vi "DPO_7K_Set_Number_of_Averages.vi"(8 "Error In":errorcluster, 10 "Number of Waveforms":i32, 11 "VISA resource name in":refnum<visa-resource-name>) -> (0 "Error Out":errorcluster, 3 "VISA resource name out":refnum<visa-resource-name>)   [LabVIEW 2020]
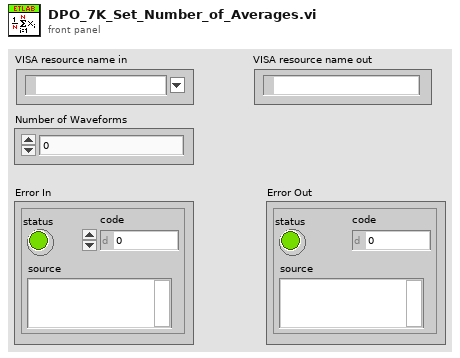
[diagram p1: front panel]
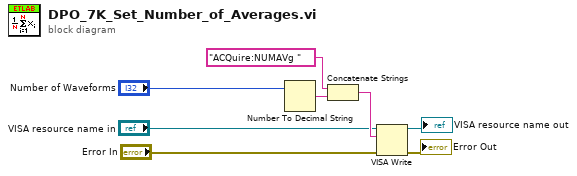
[diagram p0: block diagram]
diagram:
  n1 = Number To Decimal String(number="Number of Waveforms") -> (decimal integer string=w7:string)  [unwired: 1 in]
  n2 = Concatenate Strings("ACQuire:NUMAVg " ("write buffer"), w7) -> (w5:string)
  n3 = VISA Write(VISA resource name="VISA resource name in", write buffer=w5, error in (no error)="Error In") -> (VISA resource name out=→"VISA resource name out":refnum<visa-resource-name>, error out=→"Error Out":errorcluster)  [unwired: 1 out]
